vi "DSF.Engine.Framework.Get State.vi"(11 "Framework in":refnum<class "DSF.Engine.Framework.lvclass">) -> (2 "State":refnum<class "Framework State.lvclass">, 3 "Framework out":refnum<class "DSF.Engine.Framework.lvclass">)   [LabVIEW 2017, in "Data Sharing Framework Engine.lvlib" / "DSF.Engine.Framework.lvclass"]
uses:
  DSF.Engine.Framework.lvclass
  State/Framework State.lvclass
  DSF.Engine.Framework.lvclass/DSF.Engine.Framework.ctl
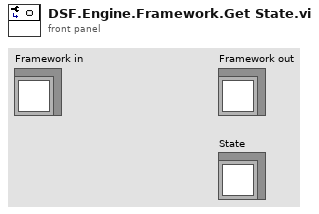
[diagram p1: front panel]
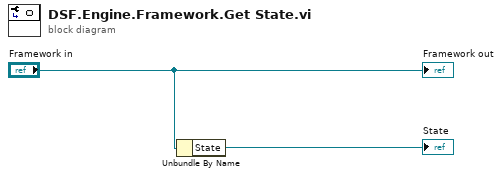
[diagram p0: block diagram]
diagram:
  n1 = Unbundle By Name("Framework in") -> ("State"=→"State":refnum<class "Framework State.lvclass">)
  "Framework out" <- "Framework in"
